vi "RLC_Domingos_Felipe_Guarnieri.vi"() -> ()   [LabVIEW 2020]
uses:
  <vilib>/Utility/file.llb/Read Delimited Spreadsheet (DBL).vi
  <vilib>/Utility/file.llb/Read Delimited Spreadsheet (string).vi
  <vilib>/ptbypt/NI_PtbyPt.lvlib
  <vilib>/gmath/NI_Gmath.lvlib
panel:
  in  "simulador":enum32{""}(tab)
  out "Entrada":cluster{dbl[], dbl[]}(graph)
  in  "on/off":bool
  in  "Tipo de Onda":u16(ring)=3 items=["Senoidal", "Quadrada", "Inserir Arquivo", "Inserir Função"]
  in  "Plot":bool caption="Teste"
  in  "Número de Amostras":dbl=10000.0
  in  "Amplitude":dbl
  in  "Frequência":dbl
  in  "Fase":dbl
  in  "Taxa de Amostragem":dbl=1000.0
  in  "Duty Cycle":dbl
  out "Saída":cluster{dbl[], dbl[]}[](graph)
  in  "Importar Arquivos":path
  in  "Vc inicial":dbl
  in  "Corrente Inicial":dbl
  in  "R":dbl=1.0
  in  "L":dbl=1.0
  in  "C":dbl=1.0
  in  "Menu Ring":u16(ring) items=["tensão", "corrente", "tensão e corrente", "entrada e saída"]
  out "?":bool
  out "Carregamento...":u8(slide) scale=0.0..100.0
  in  "Vin(t)":string="abs(ln(abs(cos(x)))) - 1"
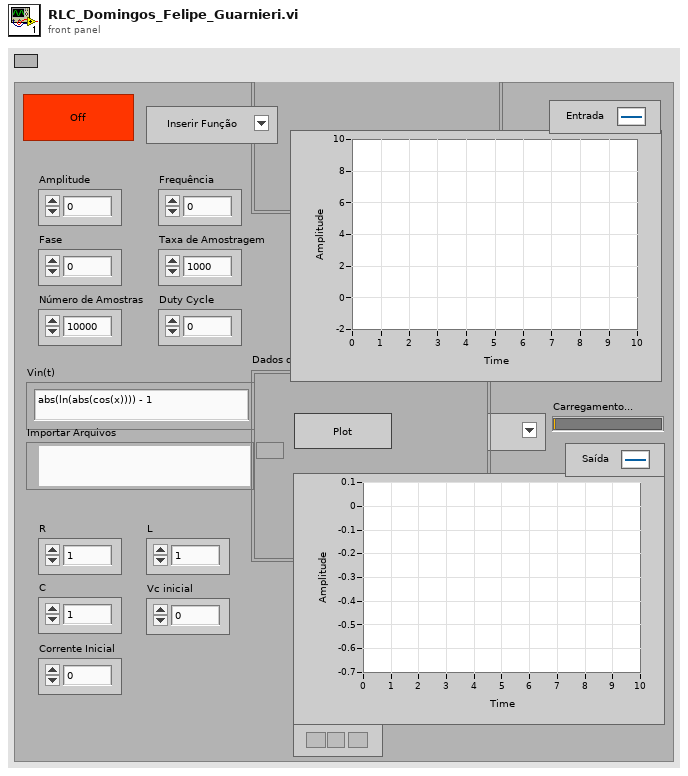
[diagram p1: front panel]
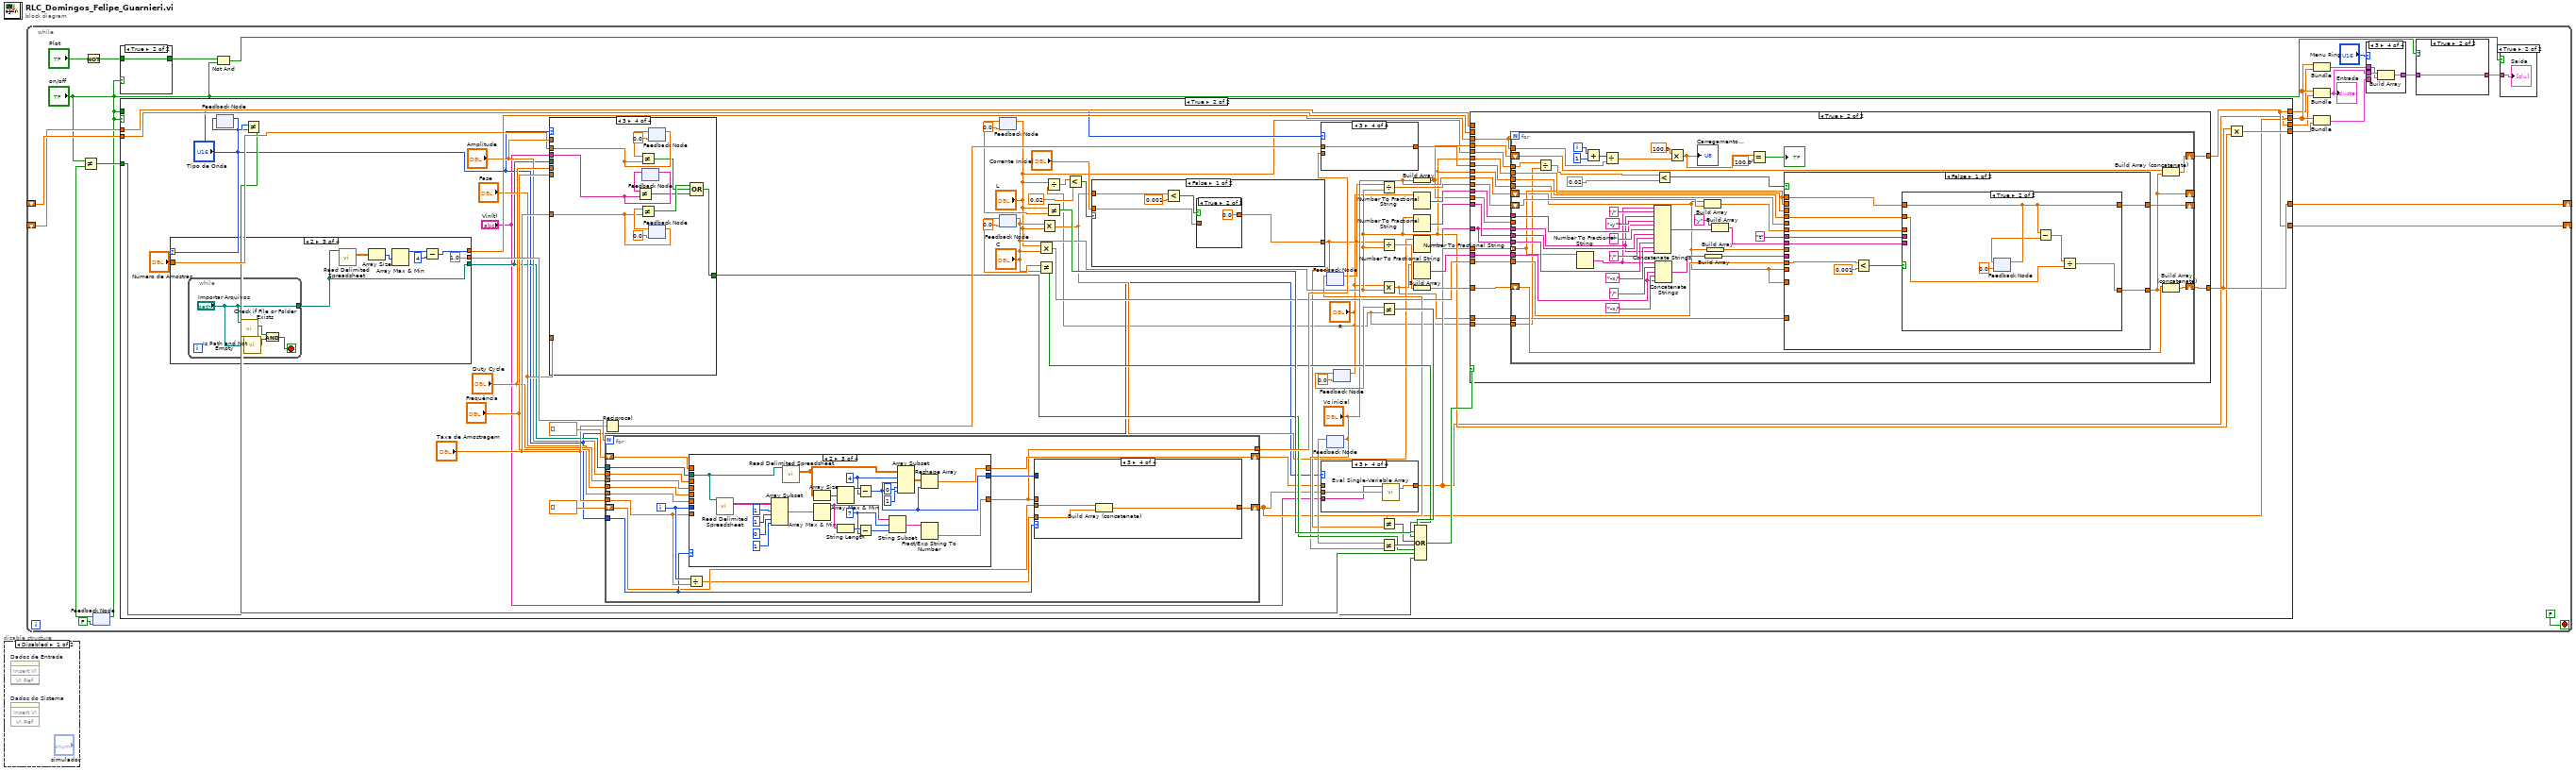
[diagram p0: block diagram]
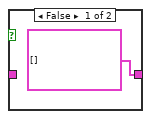
[diagram p2: hidden frame]
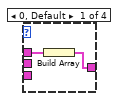
[diagram p5: hidden frame]
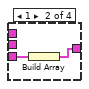
[diagram p6: hidden frame]
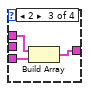
[diagram p7: hidden frame]
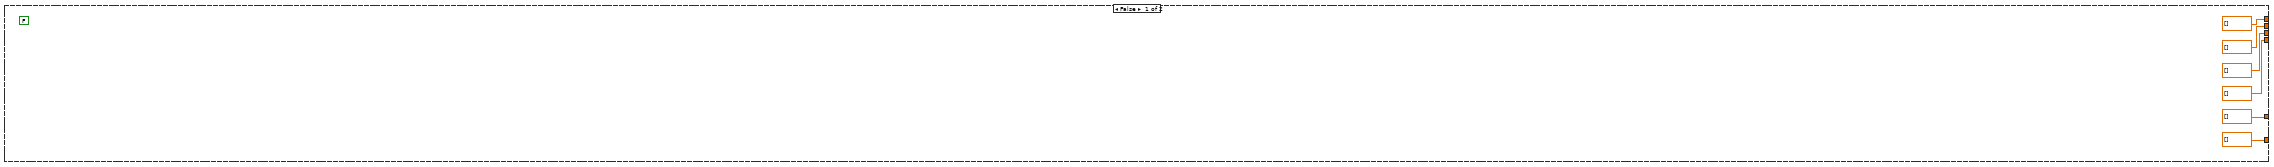
[diagram p8: hidden frame]
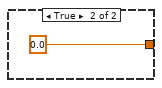
[diagram p13: hidden frame]
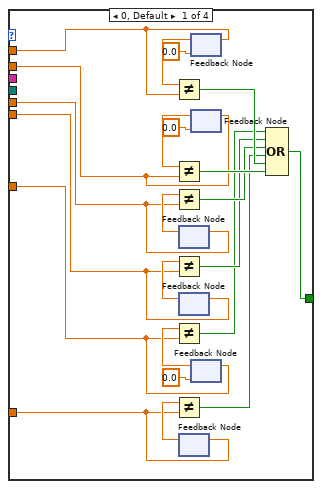
[diagram p14: hidden frame]
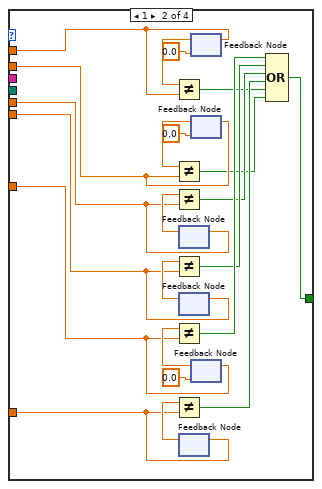
[diagram p15: hidden frame]
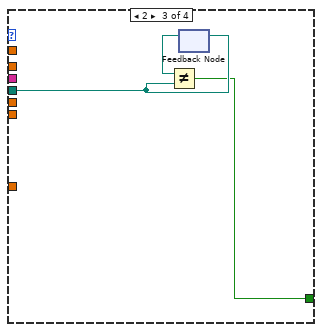
[diagram p16: hidden frame]
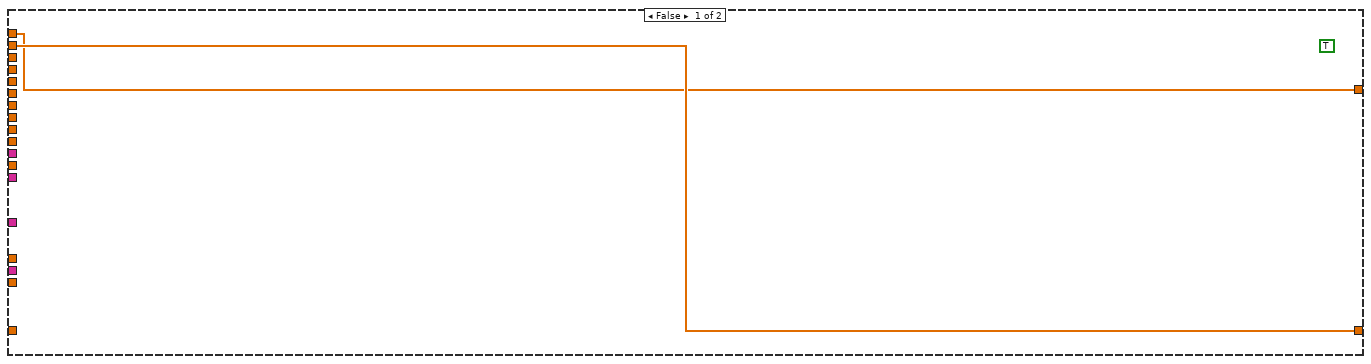
[diagram p17: hidden frame]
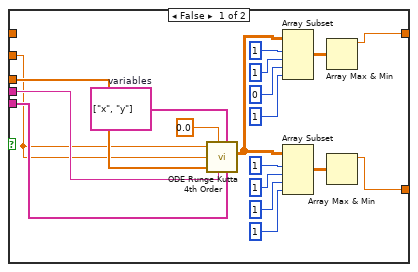
[diagram p18: hidden frame]
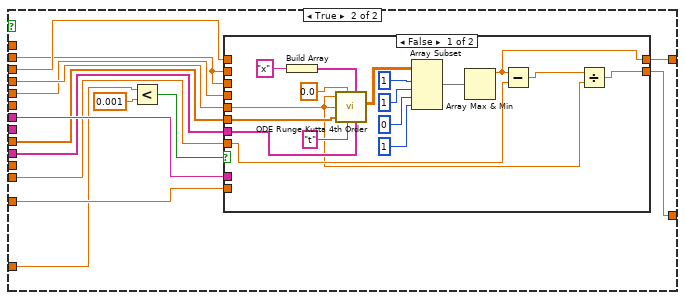
[diagram p19: hidden frame]
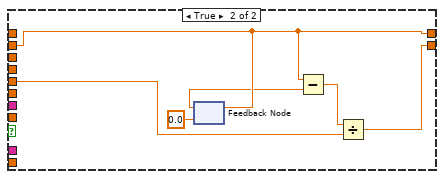
[diagram p20: hidden frame]
diagram:
  n1 = disable-structure shown="Disabled" {
    frame Disabled {
      n2 = invoke on="Dados de Entrada" class="SubPnl" method="Insert VI"() -> ()  [unwired: 4 in, 4 out]
      n3 = invoke on="Dados do Sistema" class="SubPnl" method="Insert VI"() -> ()  [unwired: 4 in, 4 out]
    }
    frame Enabled {
    }
  }
  n4 = while {
    shift-right: [w8] -> _
    shift-left: _ -> [w7]
    shift-right: [w6] -> _
    shift-left: _ -> [w5]
    stop <- FALSE stop-if-true
    n5 = Not(x="Plot") -> (.not. x?=w13:bool)
    n6 = feedback-in #1("on/off") -> ()
    n7 = feedback #1(FALSE ("on/off")) -> (w4:bool)
    n8 = Not Equal?(x="on/off", y=w4) -> (x != y?=w3:bool)
    n9 = case shown="True" "on/off" {
      selector: "on/off" -> [w26 _]
      tunnel: [w26 w27] -> w16
      tunnel: w13 -> [_ w27]
      frame False {
      }
      frame True {
      }
    }
    n10 = case shown="True" "on/off" {
      tunnel: [dbl[] [] w51] -> w22
      tunnel: [dbl[] [] w49] -> w10
      tunnel: [dbl[] [] w90] -> w9
      tunnel: [dbl[] [] w96] -> w21
      tunnel: [dbl[] [] w92] -> w8
      tunnel: w7 -> [_ w91]
      tunnel: [dbl[] [] w90] -> w6
      tunnel: w5 -> [_ w89]
      tunnel: w3 -> [_ w66]
      tunnel: "on/off" -> [_ _]
      frame False {
        (unwired) FALSE
      }
      frame True {
        n11 = case shown="2" "Tipo de Onda" {
          tunnel: [w327 w329 1.0 ("Número de Amostras") w343] -> w104
          tunnel: "Número de Amostras" -> [w327 w329 _ w343]
          tunnel: [path "" ("Importar Arquivos") path "" ("Importar Arquivos") w331 path "" ("Importar Arquivos")] -> w67
          tunnel: [w327 w329 w332 w343] -> w93
          frame 0, Default {
          }
          frame 1 {
          }
          frame 2 {
            n12 = while {
              tunnel: ["Importar Arquivos"] -> w331
              stop <- w339 stop-if-true
              n13 = call <vilib>:"Check if File or Folder Exists.vi"("path"="Importar Arquivos") -> ("file or folder exists?"=w341:bool)  [unwired: 8 in, 2 out]
              n14 = call <vilib>:"Is Path and Not Empty.vi"("path"="Importar Arquivos") -> ("Is Path and Not Empty?"=w340:bool)  [unwired: 4 in]
              n15 = And(x=w341, y=w340) -> (x .and. y?=w339:bool)
            }
            n16 = call-poly <vilib>:"Read Delimited Spreadsheet.vi"("file path (dialog if empty)"=w331) -> ("all rows"=w335:dbl[][])  [unwired: 9 in, 5 out]
            n17 = Array Size(array=w335) -> (size(s)=w337:i32[])
            n18 = Array Max & Min(array=w337) -> (max value=w336:i32)  [unwired: 3 out]
            n19 = Subtract(x=w336, y=4 ("index")) -> (x-y=w332:i32)
          }
          frame 3 {
          }
        }
        n20 = feedback-in #2("Tipo de Onda") -> ()
        n21 = feedback #2() -> (w69:u16)  [unwired: 1 in]
        n22 = Not Equal?(x=w69, y="Tipo de Onda") -> (x != y?=w68:bool)
        n23 = case shown="3" "Tipo de Onda" {
          tunnel: "Taxa de Amostragem" -> [w127 w162 _ w174]
          tunnel: "Frequência" -> [w126 w158 _ _]
          tunnel: "Duty Cycle" -> [w125 w156 _ _]
          tunnel: "Fase" -> [w124 w157 _ _]
          tunnel: "Amplitude" -> [w123 w154 _ _]
          tunnel: "Número de Amostras" -> [w122 w150 _ w173]
          tunnel: [w121 w143 w165 w171] -> w70
          tunnel: w67 -> [_ _ w166 _]
          tunnel: "Vin(t)" -> [_ _ _ w169]
          frame 0, Default {
            n24 = feedback #3() -> (w133:dbl)  [unwired: 1 in]
            n25 = Not Equal?(x=w133, y=w125) -> (x != y?=w139:bool)
            n26 = feedback-in #3(w125) -> ()
            n27 = feedback #4() -> (w132:dbl)  [unwired: 1 in]
            n28 = Not Equal?(x=w132, y=w126) -> (x != y?=w138:bool)
            n29 = feedback-in #4(w126) -> ()
            n30 = feedback #5() -> (w134:dbl)  [unwired: 1 in]
            n31 = Not Equal?(x=w134, y=w124) -> (x != y?=w140:bool)
            n32 = feedback-in #5(w124) -> ()
            n33 = feedback #6(0.0 ("Amplitude")) -> (w135:dbl)
            n34 = Not Equal?(x=w135, y=w123) -> (x != y?=w141:bool)
            n35 = feedback-in #6(w123) -> ()
            n36 = feedback #7(0.0 ("Amplitude")) -> (w136:dbl)
            n37 = Not Equal?(x=w136, y=w122) -> (x != y?=w142:bool)
            n38 = feedback-in #7(w122) -> ()
            n39 = feedback #8(0.0 ("Taxa de Amostragem")) -> (w131:dbl)
            n40 = Not Equal?(x=w131, y=w127) -> (x != y?=w137:bool)
            n41 = feedback-in #8(w127) -> ()
            n42 = Compound Arithmetic op=OR(w137, w138, w139, w140, w141, w142) -> (w121:bool)
          }
          frame 1 {
            n43 = feedback #9() -> (w160:dbl)  [unwired: 1 in]
            n44 = Not Equal?(x=w160, y=w156) -> (x != y?=w147:bool)
            n45 = feedback-in #9(w156) -> ()
            n46 = feedback #10() -> (w161:dbl)  [unwired: 1 in]
            n47 = Not Equal?(x=w161, y=w158) -> (x != y?=w148:bool)
            n48 = feedback-in #10(w158) -> ()
            n49 = feedback #11() -> (w159:dbl)  [unwired: 1 in]
            n50 = Not Equal?(x=w159, y=w157) -> (x != y?=w146:bool)
            n51 = feedback-in #11(w157) -> ()
            n52 = feedback #12(0.0 ("Amplitude")) -> (w155:dbl)
            n53 = Not Equal?(x=w155, y=w154) -> (x != y?=w145:bool)
            n54 = feedback-in #12(w154) -> ()
            n55 = feedback #13(0.0 ("Amplitude")) -> (w152:dbl)
            n56 = Not Equal?(x=w152, y=w150) -> (x != y?=w144:bool)
            n57 = feedback-in #13(w150) -> ()
            n58 = feedback #14(0.0 ("Taxa de Amostragem")) -> (w164:dbl)
            n59 = Not Equal?(x=w164, y=w162) -> (x != y?=w149:bool)
            n60 = feedback-in #14(w162) -> ()
            n61 = Compound Arithmetic op=OR(w149, w148, w147, w146, w145, w144) -> (w143:bool)
          }
          frame 2 {
            n62 = feedback-in #15(w166) -> ()
            n63 = feedback #15() -> (w167:path)  [unwired: 1 in]
            n64 = Not Equal?(x=w167, y=w166) -> (x != y?=w165:bool)
          }
          frame 3 {
            n65 = feedback-in #16(w169) -> ()
            n66 = feedback #16() -> (w170:string)  [unwired: 1 in]
            n67 = Not Equal?(x=w170, y=w169) -> (x != y?=w168:bool)
            n68 = feedback #17(0.0 ("Amplitude")) -> (w178:dbl)
            n69 = Not Equal?(x=w178, y=w173) -> (x != y?=w172:bool)
            n70 = feedback-in #17(w173) -> ()
            n71 = feedback #18(0.0 ("Taxa de Amostragem")) -> (w177:dbl)
            n72 = Not Equal?(x=w177, y=w174) -> (x != y?=w179:bool)
            n73 = feedback-in #18(w174) -> ()
            n74 = Compound Arithmetic op=OR(w179, w172, w168) -> (w171:bool)
          }
        }
        n75 = Reciprocal(x="Taxa de Amostragem") -> (1/x=w98:dbl)
        n76 = for {
          N: w104 -> [_]
          tunnel: "Taxa de Amostragem" -> [w353]
          shift-right: [w347] -> w51
          shift-left: dbl[] [] -> [w349]
          tunnel: "Tipo de Onda" -> [w350]
          tunnel: "Fase" -> [w358]
          tunnel: "Frequência" -> [w357]
          tunnel: "Amplitude" -> [w356]
          shift-right: [w351] -> w52
          shift-left: dbl[] [] -> [w352]
          tunnel: "Duty Cycle" -> [w355]
          tunnel: w67 -> [w345]
          tunnel: [w344] -> w99
          i -> [w354]
          n77 = Divide(x=w354, y=w353) -> (x/y=w348:dbl)
          n78 = case shown="2" w350 {
            tunnel: w358 -> [w385 w399 _ _]
            tunnel: w357 -> [w384 w400 _ _]
            tunnel: w356 -> [w383 w391 _ _]
            tunnel: w354 -> [w381 w401 _ _]
            tunnel: w355 -> [_ w393 _ _]
            tunnel: w353 -> [w382 w398 _ _]
            tunnel: w352 -> [w380 w397 _ _]
            tunnel: [w379 w396 w406 dbl[] []] -> w351
            tunnel: [0.0 0.0 w405 0.0] -> w344
            tunnel: [0 0 w404 0] -> w346
            tunnel: w345 -> [_ _ w403 _]
            frame 0, Default {
              n79 = Divide(x=w381, y=w382) -> (x/y=w387:dbl)
              n80 = call <vilib>:"Sine Wave PtByPt.vi"("time"=w387, "phase"=w385, "frequency"=w384, "amplitude"=w383) -> ("sine wave"=w386:dbl)
              n81 = Build Array (concatenate)(w380, w386) -> (w379:dbl[])
            }
            frame 1 {
              n82 = Divide(x=w401, y=w398) -> (x/y=w402:dbl)
              n83 = Divide(x=w391, y=2.0) -> (x/y=w390:dbl)
              n84 = call <vilib>:"Square Wave PtByPt.vi"("amplitude"=w390, "frequency"=w400, "phase"=w399, "time"=w402, "duty cycle (%)"=w393) -> ("square wave"=w389:dbl)
              n85 = Add(x=w390, y=w389) -> (x+y=w388:dbl)
              n86 = Build Array (concatenate)(w397, w388) -> (w396:dbl[])
            }
            frame 2 {
              w408 = 4 ("index")
              w416 = 7 ("offset (0)")
              n87 = call-poly <vilib>:"Read Delimited Spreadsheet.vi"("file path (dialog if empty)"=w403) -> ("all rows"=w424:string[][])  [unwired: 9 in, 5 out]
              n88 = Array Subset(array=w424, index (row)=1 ("index"), length (row)=1 ("length"), index (col)=0 ("index"), length (col)=1 ("length")) -> (w419:string[][])
              n89 = call-poly <vilib>:"Read Delimited Spreadsheet.vi"("file path (dialog if empty)"=w403) -> ("all rows"=w409:dbl[][])  [unwired: 9 in, 5 out]
              n90 = Array Size(array=w409) -> (size(s)=w413:i32[])
              n91 = Array Max & Min(array=w419) -> (max value=w418:string)  [unwired: 3 out]
              n92 = Array Max & Min(array=w413) -> (max value=w412:i32)  [unwired: 3 out]
              n93 = String Length(string=w418) -> (length=w417:i32)
              n94 = Subtract(x=w412, y=w408) -> (x-y=w404:i32)
              n95 = Subtract(x=w417, y=w416) -> (x-y=w415:i32)
              n96 = String Subset(string=w418, offset (0)=w416, length (rest)=w415) -> (substring=w414:string)
              n97 = Array Subset(array=w409, index (row)=w408, length (row)=w404, index (col)=0 ("index"), length (col)=1 ("length")) -> (w407:dbl[][])
              n98 = Reshape Array(w407, w404) -> (w406:dbl[])
              n99 = Fract/Exp String To Number(string=w414) -> (number=w405:dbl)  [unwired: 3 in, 1 out]
            }
            frame 3 {
            }
          }
          n100 = case shown="3" w350 {
            tunnel: w349 -> [w360 w364 _ w376]
            tunnel: w348 -> [w359 w363 _ w375]
            tunnel: [w361 w362 w365 w374] -> w347
            tunnel: w344 -> [_ _ w367 _]
            tunnel: w346 -> [_ _ w368 _]
            frame 0, Default {
              n101 = Build Array (concatenate)(w360, w359) -> (w361:dbl[])
            }
            frame 1 {
              n102 = Build Array (concatenate)(w364, w363) -> (w362:dbl[])
            }
            frame 2 {
              n103 = for {
                N: w368 -> [_]
                tunnel: w367 -> [w373]
                shift-right: [w370] -> w365
                shift-left: dbl[] [] -> [w369]
                i -> [w372]
                n104 = Multiply(x=w372, y=w373) -> (x*y=w371:dbl)
                n105 = Build Array (concatenate)(w369, w371) -> (w370:dbl[])
              }
            }
            frame 3 {
              n106 = Build Array (concatenate)(w376, w375) -> (w374:dbl[])
            }
          }
        }
        n107 = feedback-in #19("L") -> ()
        n108 = feedback #19(0.0 ("L")) -> (w94:dbl)
        n109 = feedback #20(0.0 ("R")) -> (w82:dbl)
        n110 = feedback-in #20("C") -> ()
        n111 = Multiply(x="L", y="C") -> (x*y=w60:dbl)
        n112 = Not Equal?(x=w82, y="C") -> (x != y?=w81:bool)
        n113 = Multiply(x="C", y="L") -> (x*y=w54:dbl)
        n114 = Divide(x="L", y="R") -> (x/y=w47:dbl)
        n115 = Not Equal?(x="L", y=w94) -> (x != y?=w84:bool)
        n116 = Less?(x=w47, y=0.02) -> (x < y?=w55:bool)
        n117 = case shown="False" w55 {
          tunnel: [w116 0.0 ("Corrente Inicial")] -> w57
          tunnel: "Corrente Inicial" -> [w117 _]
          tunnel: w54 -> [w115 _]
          frame False {
            n118 = Less?(x=w115, y=0.001) -> (x < y?=w113:bool)
            n119 = case shown="True" w113 {
              tunnel: w117 -> [w118 _]
              tunnel: [w118 0.0 ("Corrente Inicial")] -> w116
              frame False {
              }
              frame True {
              }
            }
          }
          frame True {
          }
        }
        n120 = case shown="3" "Tipo de Onda" {
          tunnel: [w323 w324 w325 w326] -> w100
          tunnel: w99 -> [_ _ w325 _]
          tunnel: w98 -> [w323 w324 _ w326]
          frame 0, Default {
          }
          frame 1 {
          }
          frame 2 {
          }
          frame 3 {
          }
        }
        n121 = case shown="3" "Tipo de Onda" {
          tunnel: [w107 w108 w109 w112] -> w49
          tunnel: w52 -> [w107 w108 w109 _]
          tunnel: w51 -> [_ _ _ w111]
          tunnel: "Vin(t)" -> [_ _ _ w110]
          frame 0, Default {
          }
          frame 1 {
          }
          frame 2 {
          }
          frame 3 {
            n122 = call <vilib>:"Eval Single-Variable Array.vi"("X Values"=w111, "formula"=w110) -> ("Y Values"=w112:dbl[])  [unwired: 1 in, 1 out]
          }
        }
        n123 = feedback #21() -> (w80:dbl)  [unwired: 1 in]
        n124 = feedback-in #21(w57) -> ()
        n125 = feedback #22() -> (w78:dbl)  [unwired: 1 in]
        n126 = feedback-in #22("Vc inicial") -> ()
        n127 = feedback-in #23("R") -> ()
        n128 = feedback #23(0.0 ("R")) -> (w87:dbl)
        n129 = Divide(x=w57, y="C") -> (x/y=w97:dbl)
        n130 = Divide(x=w57, y="C") -> (x/y=w64:dbl)
        n131 = Multiply(x="R", y="C") -> (x*y=w48:dbl)
        n132 = Not Equal?(x=w87, y="R") -> (x != y?=w86:bool)
        n133 = Not Equal?(x=w80, y=w57) -> (x != y?=w79:bool)
        n134 = Not Equal?(x=w78, y="Vc inicial") -> (x != y?=w77:bool)
        n135 = Build Array("Vc inicial") -> (w62:dbl[])
        n136 = Number To Fractional String(number="R") -> (F-format string=w103:string)  [unwired: 3 in]
        n137 = Number To Fractional String(number="C") -> (F-format string=w102:string)  [unwired: 3 in]
        n138 = Number To Fractional String(number=w54) -> (F-format string=w101:string)  [unwired: 3 in]
        n139 = Number To Fractional String(number=w48) -> (F-format string=w61:string)  [unwired: 3 in]
        n140 = Build Array(w64) -> (w63:dbl[])
        n141 = Compound Arithmetic op=OR(w86, w84, w81, w79, w77, w70, w68, w66) -> (w85:bool)
        n142 = case shown="True" w85 {
          tunnel: w103 -> [_ w201]
          tunnel: w102 -> [_ w200]
          tunnel: w101 -> [_ w199]
          tunnel: w100 -> [_ w198]
          tunnel: w49 -> [_ w197]
          tunnel: w97 -> [_ w196]
          tunnel: "Vc inicial" -> [_ w195]
          tunnel: [w181 w194] -> w92
          tunnel: w62 -> [_ w193]
          tunnel: w63 -> [_ w192]
          tunnel: [w180 w191] -> w90
          tunnel: w93 -> [_ w190]
          tunnel: w91 -> [w181 _]
          tunnel: w89 -> [w180 _]
          tunnel: w62 -> [_ w189]
          tunnel: w61 -> [_ w188]
          tunnel: "C" -> [_ w187]
          tunnel: "L" -> [_ w186]
          tunnel: w60 -> [_ w185]
          tunnel: "C" -> [_ w184]
          tunnel: w48 -> [_ w183]
          tunnel: "R" -> [_ w182]
          frame False {
            (unwired) TRUE
          }
          frame True {
            n143 = for {
              N: w190 -> [_]
              tunnel: w197 -> [w213] mode=indexing
              tunnel: w199 -> [w241]
              tunnel: w201 -> [w247]
              tunnel: w200 -> [w245]
              tunnel: w199 -> [w243]
              shift-right: [w222] -> _
              shift-left: w196 -> [w236]
              shift-right: [w221] -> _
              shift-left: w195 -> [w206]
              shift-right: [w238] -> w194
              shift-left: w192 -> [w239]
              tunnel: w198 -> [w209]
              shift-right: [w233] -> w191
              shift-left: w193 -> [w237]
              tunnel: w190 -> [w231]
              tunnel: w189 -> [_]
              tunnel: w188 -> [w217]
              tunnel: w187 -> [w214]
              tunnel: w186 -> [w204]
              tunnel: w185 -> [w210]
              tunnel: w184 -> [w207]
              tunnel: w183 -> [w205]
              tunnel: w182 -> [w203]
              i -> [w234]
              n144 = Divide(x=w204, y=w203) -> (x/y=w202:dbl)
              n145 = Number To Fractional String(number=w213) -> (F-format string=w220:string)  [unwired: 3 in]
              n146 = Add(x=w234, y=1) -> (x+y=w232:i32)
              n147 = Divide(x=w232, y=w231) -> (x/y=w230:dbl)
              n148 = Concatenate Strings(w220, "/" ("string"), w241, "-y*" ("string"), w247, "*" ("string"), w245, "/" ("string"), w243, "-x/" ("string"), w241) -> (w240:string)
              n149 = Concatenate Strings(w220, "/" ("string"), w217, "-x/" ("string"), w217) -> (w216:string)
              n150 = Less?(x=w202, y=0.02) -> (x < y?=w211:bool)
              n151 = Multiply(x=100.0, y=w230) -> (x*y=w227:dbl)
              "Carregamento..." <- w227
              n152 = Build Array(w206, w236) -> (w223:dbl[])
              n153 = Build Array(w216) -> (w215:string[])
              n154 = Build Array(w206) -> (w208:dbl[])
              n155 = Build Array("y", w240) -> (w225:string[])
              n156 = Equal?(x=w227, y=100.0) -> (x = y?=→"?":bool)
              n157 = case shown="False" w211 {
                tunnel: w225 -> [w260 _]
                tunnel: "t" -> [w259 w298]
                tunnel: w223 -> [w258 _]
                tunnel: w209 -> [w257 w299]
                tunnel: [w256 w293] -> w222
                tunnel: [w255 w296] -> w221
                tunnel: w215 -> [_ w297]
                tunnel: w214 -> [_ w295]
                tunnel: w206 -> [_ w294]
                tunnel: w213 -> [_ w290]
                tunnel: w213 -> [w254 _]
                tunnel: w210 -> [w251 _]
                tunnel: w208 -> [_ w289]
                tunnel: w207 -> [_ w288]
                tunnel: w206 -> [_ w287]
                tunnel: w205 -> [_ w286]
                frame False {
                  n158 = Less?(x=w251, y=0.001) -> (x < y?=w252:bool)
                  n159 = case shown="True" w252 {
                    tunnel: w260 -> [w279 _]
                    tunnel: w259 -> [w278 _]
                    tunnel: w258 -> [w277 _]
                    tunnel: w257 -> [w276 w281]
                    tunnel: [w262 w280] -> w256
                    tunnel: [w261 w285] -> w255
                    tunnel: w254 -> [_ w285]
                    frame False {
                      w275 = string[] ["x", "y"]  # variables
                      n160 = call <vilib>:"ODE Runge Kutta 4th Order.vi"("time end"=w276, "time start"=0.0, "h (step rate)"=w276, "X0"=w277, "time"=w278, "X (name of variables)"=w275, "F(X,t) (right sides of the ODE\nas functions of X and t)"=w279) -> ("X Values (solution)"=w263:dbl[][])  [unwired: 3 out]
                      n161 = Array Subset(array=w263, index (row)=1 ("index"), length (row)=1 ("length"), index (col)=0 ("index"), length (col)=1 ("length")) -> (w268:dbl[][])
                      n162 = Array Subset(array=w263, index (row)=1 ("index"), length (row)=1 ("length"), index (col)=1 ("index"), length (col)=1 ("length")) -> (w273:dbl[][])
                      n163 = Array Max & Min(array=w268) -> (max value=w261:dbl)  [unwired: 3 out]
                      n164 = Array Max & Min(array=w273) -> (max value=w262:dbl)  [unwired: 3 out]
                    }
                    frame True {
                      n165 = feedback-in #24(w285) -> ()
                      n166 = feedback #24(0.0 ("result")) -> (w284:dbl)
                      n167 = Subtract(x=w285, y=w284) -> (x-y=w282:dbl)
                      n168 = Divide(x=w282, y=w281) -> (x/y=w280:dbl)
                    }
                  }
                }
                frame True {
                  n169 = Less?(x=w286, y=0.001) -> (x < y?=w292:bool)
                  n170 = case shown="False" w292 {
                    tunnel: w299 -> [w302 w318]
                    tunnel: w298 -> [_ _]
                    tunnel: w297 -> [w308 _]
                    tunnel: [w304 w322] -> w296
                    tunnel: w295 -> [_ _]
                    tunnel: w294 -> [_ _]
                    tunnel: [w301 w317] -> w293
                    tunnel: w290 -> [_ w322]
                    tunnel: w290 -> [_ _]
                    tunnel: w289 -> [w307 _]
                    tunnel: w288 -> [_ _]
                    tunnel: w287 -> [w303 _]
                    frame False {
                      n171 = Build Array("x") -> (w310:string[])
                      n172 = call <vilib>:"ODE Runge Kutta 4th Order.vi"("time end"=w302, "time start"=0.0, "h (step rate)"=w302, "X0"=w307, "time"="t", "X (name of variables)"=w310, "F(X,t) (right sides of the ODE\nas functions of X and t)"=w308) -> ("X Values (solution)"=w305:dbl[][])  [unwired: 3 out]
                      n173 = Array Subset(array=w305, index (row)=1 ("index"), length (row)=1 ("length"), index (col)=0 ("index"), length (col)=1 ("length")) -> (w306:dbl[][])
                      n174 = Array Max & Min(array=w306) -> (max value=w304:dbl)  [unwired: 3 out]
                      n175 = Subtract(x=w304, y=w303) -> (x-y=w300:dbl)
                      n176 = Divide(x=w300, y=w302) -> (x/y=w301:dbl)
                    }
                    frame True {
                      n177 = feedback-in #25(w322) -> ()
                      n178 = feedback #25(0.0 ("result")) -> (w321:dbl)
                      n179 = Subtract(x=w322, y=w321) -> (x-y=w319:dbl)
                      n180 = Divide(x=w319, y=w318) -> (x/y=w317:dbl)
                    }
                  }
                }
              }
              n181 = Build Array (concatenate)(w237, w221) -> (w233:dbl[])
              n182 = Build Array (concatenate)(w239, w222) -> (w238:dbl[])
            }
          }
        }
        n183 = Multiply(x=w92, y="C") -> (x*y=w96:dbl[])
      }
    }
    n184 = Not And(1:"on/off", 2:w16) -> (0:w15:bool)
    n185 = Bundle(w22, w9) -> (w20:cluster{dbl[], dbl[]})  [unwired: 1 in]
    n186 = Bundle(w22, "Y Values"=w10) -> (w11:cluster{dbl[], "Y Values":dbl[]})  [unwired: 1 in]
    "Entrada" <- w11
    n187 = Bundle(w22, w21) -> (w19:cluster{dbl[], dbl[]})  [unwired: 1 in]
    n188 = case shown="3" "Menu Ring" {
      tunnel: w20 -> [w30 _ w33 w37]
      tunnel: [w29 w31 w35 w36] -> w17
      tunnel: w19 -> [_ w32 w34 _]
      tunnel: w11 -> [_ _ _ w38]
      frame 0, Default {
        n189 = Build Array(w30) -> (w29:cluster{dbl[], dbl[]}[])
      }
      frame 1 {
        n190 = Build Array(w32) -> (w31:cluster{dbl[], dbl[]}[])
      }
      frame 2 {
        n191 = Build Array(w33, w34) -> (w35:cluster{dbl[], dbl[]}[])
      }
      frame 3 {
        n192 = Build Array(w38, w37) -> (w36:cluster{dbl[], "Y Values":dbl[]}[])
      }
    }
    n193 = case shown="True" "on/off" {
      tunnel: [cluster{dbl[], dbl[]}[] [] w25] -> w18
      tunnel: w17 -> [_ w25]
      frame False {
      }
      frame True {
      }
    }
    n194 = case shown="True" w15 {
      tunnel: w18 -> [_ w28]
      frame False {
      }
      frame True {
        "Saída" <- w28
      }
    }
  }
